vi "Write Parameter Definition.vi"(8 "error in":errorcluster, 10 "parameter definition":T2, 11 "parameter in":T3 format="%.0x") -> (0 "error out":errorcluster, 3 "parameter out":T3 format="%.0x")   [LabVIEW 2020, in "Ballard MIL-STD-1553 Scripting.lvlib"]
uses:
  Ballard MIL-STD-1553 Scripting.lvlib
  <vilib>/NI VeriStand/Custom Device API/Custom Device Item Ref.ctl
  Shared/Parameter Definition.ctl
  Constants.vi
  <vilib>/NI VeriStand/Custom Device API/Get Item Property (String).vi
  <vilib>/NI VeriStand/Custom Device API/Get Item Property (Double).vi
  <vilib>/NI VeriStand/Custom Device API/Get Item Property (I32).vi
  <vilib>/NI VeriStand/Custom Device API/Get Item Property (U16).vi
  <vilib>/NI VeriStand/Custom Device API/Get Item Property (Boolean).vi
  <vilib>/NI VeriStand/Custom Device API/Custom Device API.lvlib
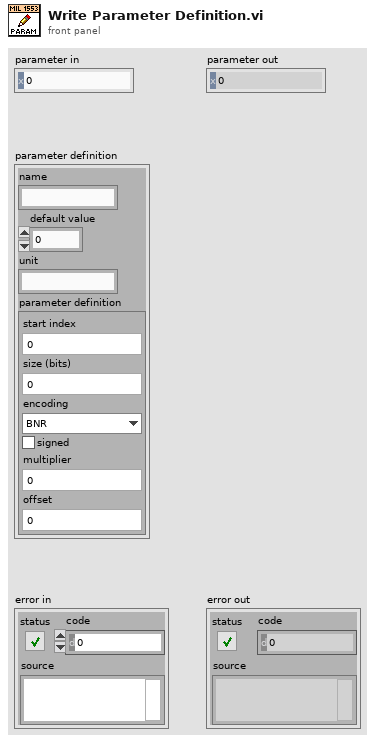
[diagram p1: front panel]
types:
  T1 = typedef "Parameter Definition.ctl" = cluster{"start index":i32, "size (bits)":i32, "encoding":enum16{"BNR", "BCD", "Discrete"}, "signed":bool, "multiplier":dbl, "offset":dbl}
  T2 = cluster{"name":string, "default value":dbl, "unit":string, "parameter definition":T1}
  T3 = typedef "Custom Device API.lvlib/Custom Device Item Ref.ctl" = u64
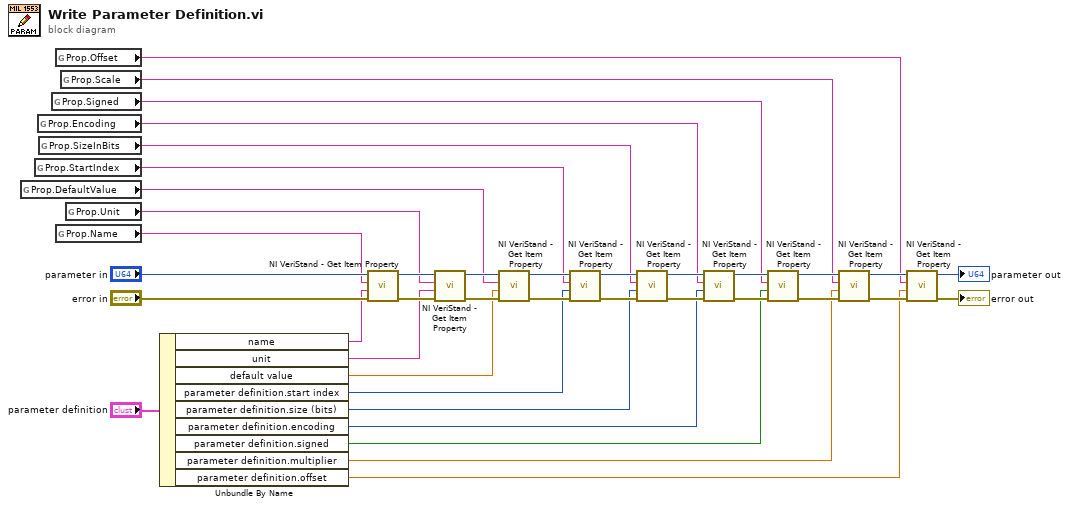
[diagram p0: block diagram]
diagram:
  n1 = global read "Constants.vi" "Prop.DefaultValue"() -> (w13:string)
  n2 = global read "Constants.vi" "Prop.StartIndex"() -> (w14:string)
  n3 = global read "Constants.vi" "Prop.Encoding"() -> (w16:string)
  n4 = global read "Constants.vi" "Prop.SizeInBits"() -> (w15:string)
  n5 = global read "Constants.vi" "Prop.Signed"() -> (w17:string)
  n6 = global read "Constants.vi" "Prop.Offset"() -> (w19:string)
  n7 = global read "Constants.vi" "Prop.Name"() -> (w12:string)
  n8 = global read "Constants.vi" "Prop.Scale"() -> (w18:string)
  n9 = global read "Constants.vi" "Prop.Unit"() -> (w11:string)
  n10 = Unbundle By Name("parameter definition") -> ("name"=w9:string, "unit"=w8:string, "default value"=w7:dbl, "parameter definition.start index"=w6:i32, "parameter definition.size (bits)"=w5:i32, "parameter definition.encoding"=w4:enum16{"BNR", "BCD", "Discrete"}, "parameter definition.signed"=w3:bool, "parameter definition.multiplier"=w2:dbl, "parameter definition.offset"=w1:dbl)
  n11 = call-poly <vilib>:"NI VeriStand - Get Item Property.vi"("error in (no error)"="error in", "Default Value"=w9, "Property Name"=w12, "Item Ref in"="parameter in") -> ("error out"=w38:errorcluster, "Item Ref out"=w39:T3)  [unwired: 4 in, 2 out]
  n12 = call-poly <vilib>:"NI VeriStand - Get Item Property.vi"("error in (no error)"=w38, "Default Value"=w8, "Property Name"=w11, "Item Ref in"=w39) -> ("error out"=w36:errorcluster, "Item Ref out"=w37:T3)  [unwired: 4 in, 2 out]
  n13 = call-poly <vilib>:"NI VeriStand - Get Item Property.vi"("error in (no error)"=w36, "Default Value"=w7, "Property Name"=w13, "Item Ref in"=w37) -> ("error out"=w34:errorcluster, "Item Ref out"=w35:T3)  [unwired: 4 in, 2 out]
  n14 = call-poly <vilib>:"NI VeriStand - Get Item Property.vi"("error in (no error)"=w34, "Default Value"=w6, "Property Name"=w14, "Item Ref in"=w35) -> ("error out"=w32:errorcluster, "Item Ref out"=w33:T3)  [unwired: 4 in, 2 out]
  n15 = call-poly <vilib>:"NI VeriStand - Get Item Property.vi"("error in (no error)"=w32, "Default Value"=w5, "Property Name"=w15, "Item Ref in"=w33) -> ("error out"=w30:errorcluster, "Item Ref out"=w31:T3)  [unwired: 4 in, 2 out]
  n16 = call-poly <vilib>:"NI VeriStand - Get Item Property.vi"("error in (no error)"=w30, "Default Value"=w4, "Property Name"=w16, "Item Ref in"=w31) -> ("error out"=w28:errorcluster, "Item Ref out"=w29:T3)  [unwired: 4 in, 2 out]
  n17 = call-poly <vilib>:"NI VeriStand - Get Item Property.vi"("error in (no error)"=w28, "Default Value"=w3, "Property Name"=w17, "Item Ref in"=w29) -> ("error out"=w26:errorcluster, "Item Ref out"=w27:T3)  [unwired: 4 in, 2 out]
  n18 = call-poly <vilib>:"NI VeriStand - Get Item Property.vi"("error in (no error)"=w26, "Default Value"=w2, "Property Name"=w18, "Item Ref in"=w27) -> ("error out"=w24:errorcluster, "Item Ref out"=w25:T3)  [unwired: 4 in, 2 out]
  n19 = call-poly <vilib>:"NI VeriStand - Get Item Property.vi"("error in (no error)"=w24, "Default Value"=w1, "Property Name"=w19, "Item Ref in"=w25) -> ("error out"=→"error out":errorcluster, "Item Ref out"=→"parameter out":T3)  [unwired: 4 in, 2 out]
